vi "IMAQDevice.startAcquisition.vi"(0 "i ref in":refnum<vi>, 5 "error in (no error)":errorcluster) -> (14 "i ref out":refnum<vi>, 19 "error out":errorcluster)   [LabVIEW 2014, in "IMAQDevice.lvlib"]
doc: "This VI starts the aqcuisition in the continous mode.\n\nLicense Agreement for this software:\n\nCopyright (C)\nGesellschaft für Schwerionenforschung, GSI\nPlanckstr. 1\n64291 Darmstadt\nGermany\n\nContact: D.Beck@gsi.de \n\nThis program is free software; you can redistribute it and/or modify it under the terms of the \nGNU General Public License as published by the Free Software Foundation; either version 2 of \nthe license, or (at your option) any later version.\n\nThis program is distributed in the hope that it will be useful, but WITHOUT ANY WARRANTY; \nwithout even the implied warranty of MERCHANTABILITY or FITNESS FOR A PARTICULAR PURPOSE. See the GNU General License for more details (http://www.gnu.org).\n\nGesellschaft für Schwerionenforschung, GSI\nPlanckstr. 1, 64291 Darmstadt, Germany\nFor all questions and ideas contact: M.Richter@gsi.de, H.Brand@gsi.de or D.Beck@gsi.de.\nLast update: 16-JUN-2004"
uses:
  IMAQDevice.lvlib
  CSlibraries-extern/HGF/HGF_LVC/HGF_IMAQ/HGF_IMAQDevice/HGF_IMAQDevice.lvclass
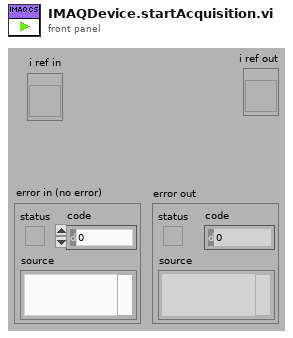
[diagram p1: front panel]
types:
  T1 = typedef "IMAQDevice.lvlib/IMAQDevice.i attribute.ctl" = cluster{"HGF_IMAQ.lvlib:HGF_IMAQDevice.lvclass":refnum<class "HGF_IMAQDevice.lvclass">, "Image":T2, "TimeStampID":i32, "Image IDs":i32[], "NumberOfImagesID":i32, "JPEG?":bool, "JPEGID":i32, "JPEG_ImageID":i32, "TriggerModeID":i32, "OffsetFromLeft":i32, "OffsetFromTop":i32, "HorizontalPixelPerMm":dbl, "VerticalPixelPerMm":dbl, "Grid":cluster{"1":cluster{i32, i32}, "2":cluster{i32, i32}, "3":cluster{i32, i32}, "4":cluster{i32, i32}}, "GridR":cluster{"1":cluster{dbl, dbl}, "2":cluster{dbl, dbl}, "3":cluster{dbl, dbl}, "4":cluster{dbl, dbl}}, "CameraTypeID":i32, "CameraInfos":cluster{"Camera Name-Array":string[], "own Camera Type":string}, "TakeMeasurement?":bool, "TriggerArmedID":i32, "Mirroring":i16, "Rotation":dbl}
  T2 = typedef "IMAQ Image.ctl" = refnum<image>
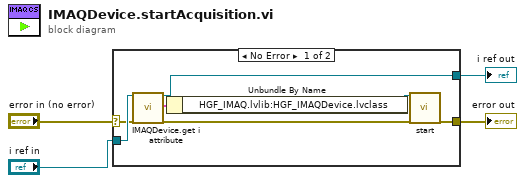
[diagram p0: block diagram]
diagram:
  n1 = case shown="No Error" "error in (no error)" {
    selector: "error in (no error)" -> [w10 w13]
    tunnel: "i ref in" -> [w11 w12]
    tunnel: [w7 w13] -> w2
    tunnel: [w9 w12] -> w1
    frame No Error {
      n2 = call "IMAQDevice.get i attribute.vi"("i ref in"=w11, "error in (no error)"=w10) -> ("i ref out"=w9:refnum<vi>, "i attribute"=w8:T1, "error out"=w6:errorcluster)  [unwired: 15 in]
      n3 = Unbundle By Name(w8) -> ("HGF_IMAQ.lvlib:HGF_IMAQDevice.lvclass"=w5:refnum<class "HGF_IMAQDevice.lvclass">)
      n4 = call "start.vi"("HGF_IMAQDevice"=w5, "error in (no error)"=w6) -> ("error out"=w7:errorcluster)  [unwired: 16 in, 1 out]
    }
    frame Error {
    }
  }
  "i ref out" <- w1
  "error out" <- w2
